vi "ShowHistoryGraph.vi"(8 "error in":errorcluster caption="错误输入（无错误）", 11 "PCM MenuVIPanelSplit.lvclass":refnum<class "PCM MenuVIPanelSplit.lvclass">) -> (0 "error out":errorcluster caption="错误输出", 3 "PCM MenuVIPanelSplit.lvclass out":refnum<class "PCM MenuVIPanelSplit.lvclass">)   [LabVIEW 2016, in "PCM MenuVIPanelSplit.lvclass"]
uses:
  PCM MenuVIPanelSplit.lvclass
  C:/Users/CL/Desktop/ZcDAQprj0811/ZcDAQprj/Modules/DAQ-Display/PanelSplitToolkit/PanelRootNode/PanelRootNode.lvclass
  PanelSplitToolkit/PanelRootNode/PanelRootNode.lvclass
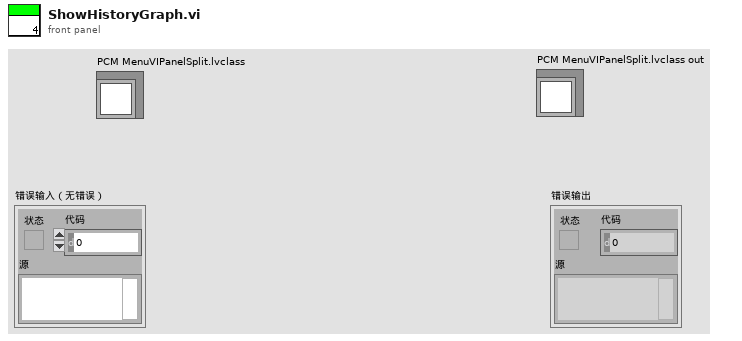
[diagram p1: front panel]
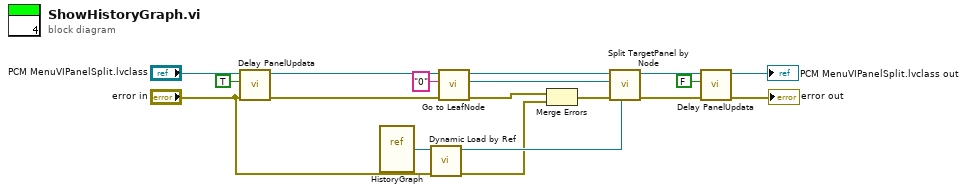
[diagram p0: block diagram]
diagram:
  n1 = call "Delay PanelUpdata.vi"("error in"="error in", "延迟前面板更新"=TRUE, "PanelRootNode 输入"="PCM MenuVIPanelSplit.lvclass") -> ("error out"=w13:errorcluster, "PanelRootNode 输出"=w1:refnum<class "PCM MenuVIPanelSplit.lvclass">)  [unwired: 7 in]
  n2 = vi-ref "HistoryGraph.vi"() -> (w14:refnum<vi>)
  n3 = call "Dynamic Load by Ref.vi"("error in"="error in", "Static vi reference in"=w14) -> ("错误输出"=w3:errorcluster, "Dynamic vi reference out"=w15:refnum<vi>)  [unwired: 8 in]
  n4 = call-dynamic "Go to LeafNode.vi"("error in"=w13, "LeafNumber"="0", "PanelRootNode 输入"=w1) -> ("error out"=w4:errorcluster, "Node*"=w17:refnum<data-value>, "PanelRootNode 输出"=w18:refnum<class "PCM MenuVIPanelSplit.lvclass">)  [unwired: 5 in, 1 out]
  n5 = Merge Errors(w4, w3) -> (w2:errorcluster)
  n6 = call-dynamic "Split TargetPanel by Node.vi"("Dynamic VI*"=w15, "error in"=w2, "Node*"=w17, "PanelRootNode 输入"=w18) -> ("error out"=w10:errorcluster, "PanelRootNode 输出"=w9:refnum<class "PCM MenuVIPanelSplit.lvclass">)  [unwired: 5 in, 1 out]
  n7 = call "Delay PanelUpdata.vi"("error in"=w10, "延迟前面板更新"=FALSE, "PanelRootNode 输入"=w9) -> ("error out"=→"error out":errorcluster, "PanelRootNode 输出"=→"PCM MenuVIPanelSplit.lvclass out":refnum<class "PCM MenuVIPanelSplit.lvclass">)  [unwired: 7 in]
